vi "SRV_Write System Config File.vi"(0 "System Config File Path":path, 7 "System Config":T1={"SRV IP Address"="", "Video Stream Rate Period (ms)"=250, "Enable Diagnostic Log"=FALSE, "Watchdog 1 Config"={"Watchdog Name"="", "Watchdog Period (s)"=1.0, "Watchdog Command"={"I2C Address"=0, "Register"=0, "Value"=0, "Active"=FALSE}}, "Watchdog 2 Config"={"Watchdog Name"="", "Watchdog Period (s)"=1.0, "Watchdog Command"={"I2C Address"=0, "Register"=0, "Value"=0, "Active"=FALSE}}, "Sensor Window Filepath"=path ""} {"Watchdog 2 Config"."Watchdog Period (s)" format="%.3f"; "Watchdog 2 Config"."Watchdog Command"."Value" format="%02x"; "Watchdog 2 Config"."Watchdog Command"."Register" format="%02x"; "Watchdog 2 Config"."Watchdog Command"."I2C Address" format="%02x"; "Watchdog 1 Config"."Watchdog Period (s)" format="%.3f"; "Watchdog 1 Config"."Watchdog Command"."Value" format="%02x"; "Watchdog 1 Config"."Watchdog Command"."Register" format="%02x"; "Watchdog 1 Config"."Watchdog Command"."I2C Address" format="%02x"}, 11 "error in (no error)":errorcluster) -> (15 "error out":errorcluster)   [LabVIEW 2014]
uses:
  SRV_System Config.ctl
  Watchdog/SRV_Watchdog Config Cluster.ctl
  Motors/Motors Config/SRV_Motor Control Command Config.ctl
  <vilib>/Utility/xml.llb/Write to XML File(string).vi
panel:
  # "I2C Address"
  # "Register"
  # "Value"
  # "Active"
  # "I2C Address"
  # "Register"
  # "Value"
  # "Active"
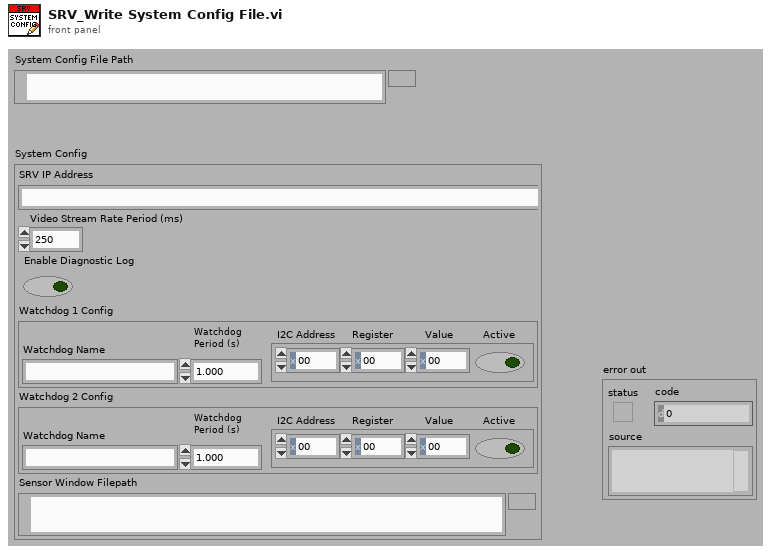
[diagram p1: front panel]
types:
  T1 = typedef "SRV_System Config.ctl" = cluster{"SRV IP Address":string, "Video Stream Rate Period (ms)":u32, "Enable Diagnostic Log":bool, "Watchdog 1 Config":T2, "Watchdog 2 Config":T2, "Sensor Window Filepath":path}
  T2 = typedef "SRV_Watchdog Config Cluster.ctl" = cluster{"Watchdog Name":string, "Watchdog Period (s)":dbl, "Watchdog Command":T3}
  T3 = typedef "SRV_Motor Control Command Config.ctl" = cluster{"I2C Address":u8, "Register":u8, "Value":u8, "Active":bool}
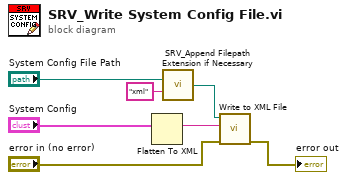
[diagram p0: block diagram]
diagram:
  n1 = Flatten To XML(anything="System Config") -> (xml string=w7:string)
  n2 = call "SRV_Append Filepath Extension if Necessary.vi"("Filepath"="System Config File Path", "Extension"="xml") -> ("Filepath with Extension"=w5:path)  [unwired: 13 in]
  n3 = call-poly <vilib>:"Write to XML File.vi"("error in (no error)"="error in (no error)", "XML Input"=w7, "XML File Path"=w5) -> ("error out"=→"error out":errorcluster)  [unwired: 6 in, 2 out]
